vi "MotorMoveIRL.vi"(11 "Rbt Cmd":string) -> (0 "error out":errorcluster)   [LabVIEW 2019]
doc: "Initializes the signals to move the designated motor in the correct direction"
uses:
  <vilib>/myRIO/Instrument Drivers/Onboard IO/DIO/typedefs/DIO Reference.ctl
  <vilib>/myRIO/Common/Instrument Driver Framework/Utilities/typedefs/myRIO Generic Hardware Reference.ctl
  <vilib>/myRIO/Common/Instrument Driver Framework/Utilities/typedefs/Hardware Version Enum.ctl
  <vilib>/myRIO/Common/Instrument Driver Framework/Utilities/typedefs/myRIO v1.0 Reference.ctl
  <vilib>/myRIO/Common/Instrument Driver Framework/Utilities/typedefs/Generic FPGA Reference.ctl
  <vilib>/myRIO/Common/Instrument Driver Framework/myRIO v1.0/DIO/typedefs/DIO Channels List.ctl
  <vilib>/myRIO/Common/Instrument Driver Framework/myRIO v1.0/DIO/typedefs/DIO Channels Enum.ctl
  <vilib>/userDefined/High Color/nirio_resource_hc.ctl
  <vilib>/myRIO/Instrument Drivers/Onboard IO/AO/typedefs/AO Reference.ctl
  <vilib>/myRIO/Common/Instrument Driver Framework/myRIO v1.0/AO/typedefs/AO Channels List.ctl
  <vilib>/myRIO/Common/Instrument Driver Framework/myRIO v1.0/AO/typedefs/AO Channels Enum.ctl
  <vilib>/myRIO/Common/Instrument Driver Framework/Utilities/typedefs/Analog Scaling Constants List.ctl
  <vilib>/myRIO/Common/Instrument Driver Framework/Utilities/typedefs/Analog Scaling Constants.ctl
  <vilib>/myRIO/Common/Instrument Driver Framework/myRIO v1.0/Encoder/typedefs/Encoder Signal Mode.ctl
  <vilib>/myRIO/Instrument Drivers/Onboard IO/Encoder/typedefs/Encoder Reference.ctl
  <vilib>/myRIO/Common/Instrument Driver Framework/myRIO v1.0/Encoder/typedefs/Encoder Channels Enum.ctl
  <vilib>/myRIO/Common/Instrument Driver Framework/myRIO v1.0/Encoder/typedefs/Encoder Configuration v1.0.ctl
  <vilib>/myRIO/Common/Instrument Driver Framework/Utilities/vis/Is FPGA Ref Available.vi
  <vilib>/myRIO/Common/Instrument Driver Framework/myRIO v1.0/DIO/vis/myRIO v1.1 Open DIO.vi
  <vilib>/myRIO/Instrument Drivers/Onboard IO/DIO/vis/Write.vi
  <vilib>/myRIO/Common/Instrument Driver Framework/myRIO v1.0/AO/vis/myRIO v1.1 Open AO.vi
  <vilib>/myRIO/Instrument Drivers/Onboard IO/AO/vis/Write.vi
  <vilib>/myRIO/Common/Instrument Driver Framework/myRIO v1.0/Encoder/vis/myRIO v1.1 Open Encoder.vi
  <vilib>/myRIO/Instrument Drivers/Onboard IO/Encoder/vis/Read.vi
  <vilib>/myRIO/Common/Instrument Driver Framework/Utilities/vis/Validate Channels.vi
  <vilib>/myRIO/Common/Instrument Driver Framework/myRIO v1.0/DIO/vis/myRIO v1.0 Reserve DIO.vi
  <vilib>/myRIO/Common/Instrument Driver Framework/myRIO v1.0/AO/vis/myRIO v1.0 Reserve AO.vi
  <vilib>/myRIO/Common/Instrument Driver Framework/myRIO v1.0/Encoder/vis/myRIO v1.0 Reserve Encoder.vi
  <vilib>/myRIO/Common/Instrument Driver Framework/myRIO v1.0/Resource Manager/vis/myRIO v1.0 Reserve Channel List.vi
  <vilib>/myRIO/Common/Instrument Driver Framework/myRIO v1.0/DIO/vis/myRIO v1.0 Build MUX Configuration DIO.vi
  <vilib>/myRIO/Common/Instrument Driver Framework/myRIO v1.0/AO/vis/myRIO v1.0 Build MUX Configuration AO.vi
  <vilib>/myRIO/Common/Instrument Driver Framework/myRIO v1.0/Encoder/vis/myRIO v1.0 Build MUX Configuration Encoder.vi
  <vilib>/myRIO/Common/Instrument Driver Framework/myRIO v1.0/Resource Manager/vis/myRIO v1.0 Reserve Channel.vi
  <vilib>/myRIO/Common/Instrument Driver Framework/myRIO v1.0/Resource Manager/vis/myRIO v1.0 Unreserve Channel.vi
  <vilib>/myRIO/Common/Instrument Driver Framework/myRIO v1.0/Resource Manager/vis/myRIO v1.0 Create Configuration List.vi
  <vilib>/myRIO/Common/Instrument Driver Framework/myRIO v1.0/Resource Manager/vis/myRIO v1.0 Build Mutex Name.vi
  <vilib>/Utility/VariantDataType/GetNumericInfo.vi
  <vilib>/Utility/error.llb/Error Cluster From Error Code.vi
  <vilib>/myRIO/Common/Instrument Driver Framework/myRIO v1.0/myRIO v1.1 Open.vi
  <vilib>/myRIO/Common/Instrument Driver Framework/Utilities/vis/IO Manager.vi
  <vilib>/myRIO/Common/Instrument Driver Framework/Utilities/vis/Configuration Manager.vi
  <vilib>/myRIO/Common/Instrument Driver Framework/myRIO v1.0/Resource Manager/vis/myRIO v1.0 Configure IO.vi
  <vilib>/myRIO/Common/Instrument Driver Framework/myRIO v1.0/myRIO v1.0 Close.vi
  <vilib>/myRIO/Common/Instrument Driver Framework/myRIO v1.0/DIO/vis/myRIO v1.0 Write DIO.vi
  <vilib>/myRIO/Common/Instrument Driver Framework/myRIO v1.0/AO/vis/myRIO v1.0 Get Scaling Constants AO.vi
  <vilib>/myRIO/Common/Instrument Driver Framework/myRIO v1.0/AO/vis/myRIO v1.0 Write AO.vi
  <vilib>/myRIO/Common/Instrument Driver Framework/myRIO v1.0/Encoder/vis/myRIO v1.0 Configure Encoder.vi
  <vilib>/myRIO/Common/Instrument Driver Framework/myRIO v1.0/Encoder/vis/myRIO v1.0 Read Encoder.vi
  <vilib>/myRIO/Express VI/Onboard IO/DO/DO Express VI.xnode
  <vilib>/myRIO/Instrument Drivers/Onboard IO/DIO/vis/myRIO DIO Open.xnode
  <vilib>/myRIO/Express VI/Onboard IO/AO/AO Express VI.xnode
  <vilib>/myRIO/Instrument Drivers/Onboard IO/AO/vis/myRIO AO Open.xnode
  <vilib>/myRIO/Express VI/Onboard IO/Encoder/Encoder Express VI.xnode
  <vilib>/myRIO/Instrument Drivers/Onboard IO/Encoder/vis/myRIO Encoder Open.xnode
  <vilib>/myRIO/Common/Instrument Driver Framework/myRIO v1.0/Encoder/typedefs/Encoder Count Direction Enum.ctl
  <vilib>/myRIO/Instrument Drivers/Onboard IO/Encoder/Encoder.lvlib
  <vilib>/myRIO/Instrument Drivers/Onboard IO/DIO/DIO.lvlib
  <vilib>/myRIO/Instrument Drivers/Onboard IO/AO/AO.lvlib
panel:
  out "Enco B'":i32
  out "Enco R'":i32
  out "Enco L'":i32
  out "Enco F'":i32
  out "Enco D'":i32
  out "Enco U'":i32
  out "Enco D":i32
  out "Enco U":i32
  out "Enco B":i32
  out "Enco R":i32
  out "Enco L":i32
  out "Enco F":i32
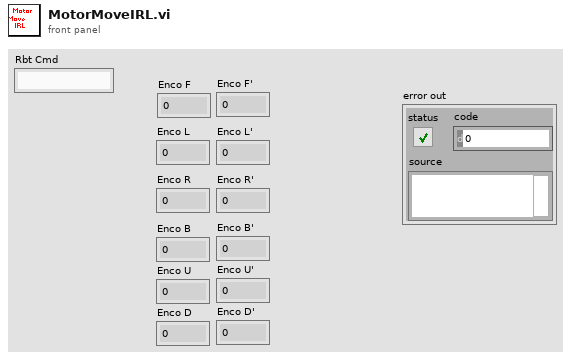
[diagram p1: front panel]
types:
  T1 = typedef "AO.lvlib/AO Reference.ctl" = cluster{"myRIO Reference":T2, "AO Channel List":T6, "AO Scaling Constant List":T8}
  T2 = typedef "myRIO Generic Hardware Reference.ctl" = cluster{"myRIO Model":T3, "myRIO Hardware Reference":T4}
  T3 = typedef "Hardware Version Enum.ctl" = enum16{"Unknown", "myRIO-1900", "myRIO-1950", "roboRIO", "NI ELVIS RIO CM", "ELVIS III"}
  T4 = typedef "myRIO v1.0 Reference.ctl" = cluster{"Generic FPGA Reference":T5, "Allow multiple opens":bool}
  T5 = typedef "Generic FPGA Reference.ctl" = refnum<k20>
  T6 = typedef "AO Channels List.ctl" = T7[]
  T7 = typedef "AO Channels Enum.ctl" = enum16{"Not Connected", "AudioOut/Left", "AudioOut/Right", "C/AO0", "C/AO1", "A/AO0", "A/AO1", "B/AO0", "B/AO1"}
  T8 = typedef "Analog Scaling Constants List.ctl" = T9[]
  T9 = typedef "Analog Scaling Constants.ctl" = cluster{"LSB Weight (Volts)":dbl, "Offset (Volts)":dbl, "Signed?":bool}
  T10 = typedef "nirio_resource_hc.ctl" = tag
  T11 = typedef "Encoder.lvlib/Encoder Reference.ctl" = cluster{"myRIO Reference":T2, "Encoder Channels Enum":T12}
  T12 = typedef "Encoder Channels Enum.ctl" = enum16{"Not Connected", "C/ENC0", "C/ENC1", "A/ENC", "A/ENC0", "A/ENC1", "A/ENC2", "A/ENC3", "A/ENC4", "A/ENC5", "A/ENC6", "A/ENC7", "A/ENC8", "A/ENC9", "B/ENC", "B/ENC0", "B/ENC1", "B/ENC2", "B/ENC3", "B/ENC4", "B/ENC5", "B/ENC6", "B/ENC7", "B/ENC8", "B/ENC9", "DIO/ENC0", "DIO/ENC1", "DIO/ENC2", "DIO/ENC3", "DIO/ENC4"}
  T13 = typedef "Encoder Signal Mode.ctl" = enum16{"Quadrature phase signal", "Step and direction signal"}
  T14 = typedef "DIO.lvlib/DIO Reference.ctl" = cluster{"myRIO Reference":T2, "DIO Channels List":T15}
  T15 = typedef "DIO Channels List.ctl" = T16[]
  T16 = typedef "DIO Channels Enum.ctl" = enum16{"Not Connected", "C/DIO0", "C/DIO1", "C/DIO2", "C/DIO3", "C/DIO4", "C/DIO5", "C/DIO6", "C/DIO7", "A/DIO0", "A/DIO1", "A/DIO2", "A/DIO3", "A/DIO4", "A/DIO5", "A/DIO6", "A/DIO7", "A/DIO8", "A/DIO9", "A/DIO10", "A/DIO11", "A/DIO12", "A/DIO13", "A/DIO14", "A/DIO15", "A/DIO16", "A/DIO17", "A/DIO18", "A/DIO19", "B/DIO0", "B/DIO1", "B/DIO2", "B/DIO3", "B/DIO4", "B/DIO5", "B/DIO6", "B/DIO7", "B/DIO8", "B/DIO9", "B/DIO10", "B/DIO11", "B/DIO12", "B/DIO13", "B/DIO14", "B/DIO15", "B/DIO16", "B/DIO17", "B/DIO18", "B/DIO19", "LED0", "LED1", "LED2", "LED3", "Button0", "DIO/DIO0", "DIO/DIO1", "DIO/DIO2", "DIO/DIO3", "DIO/DIO4", "DIO/DIO5", "DIO/DIO6", "DIO/DIO7", "DIO/DIO8", "DIO/DIO9", "SPI/CS0", "SPI/CS1", "SPI/CS2", "SPI/CS3", "LED RADIO (Green)", "LED RADIO (Red)", "LED COMM (Green)", "LED COMM (Red)", "LED MODE (Green)", "LED MODE (Red)"}
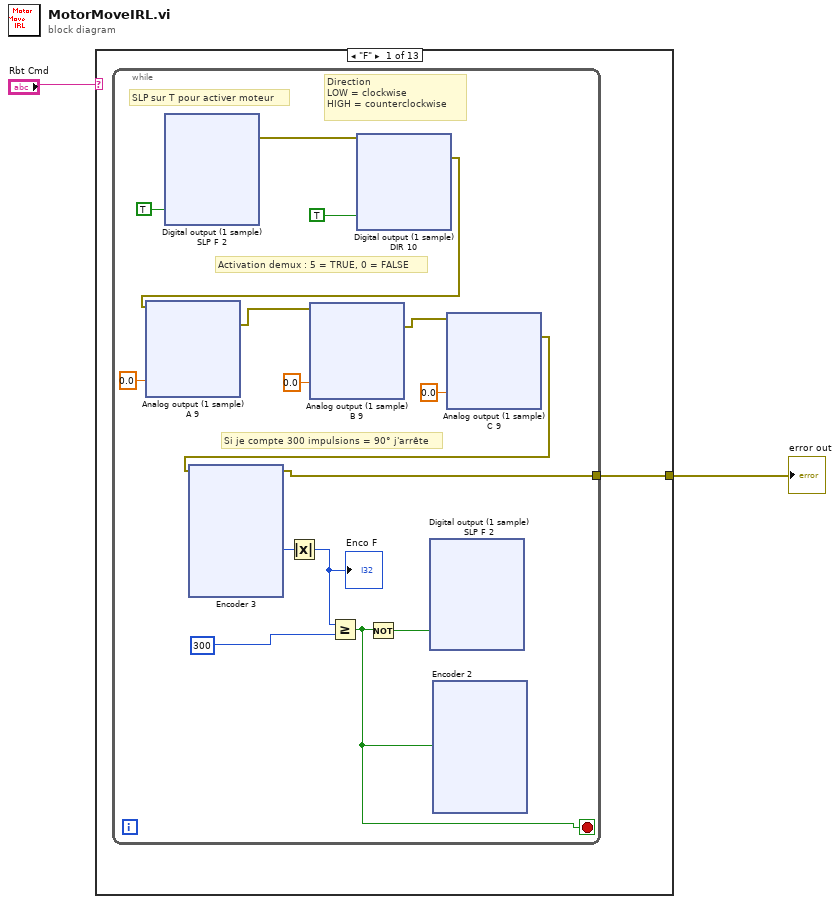
[diagram p0: block diagram]
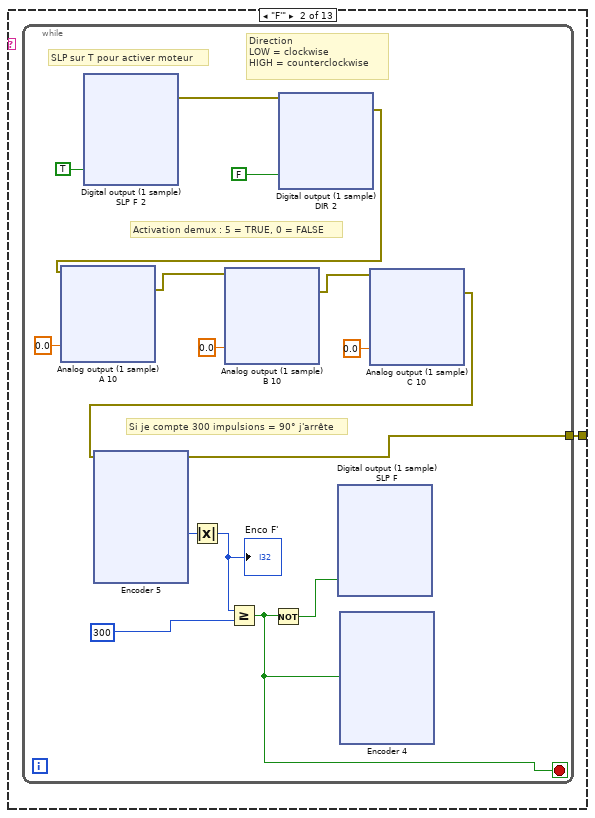
[diagram p2: hidden frame]
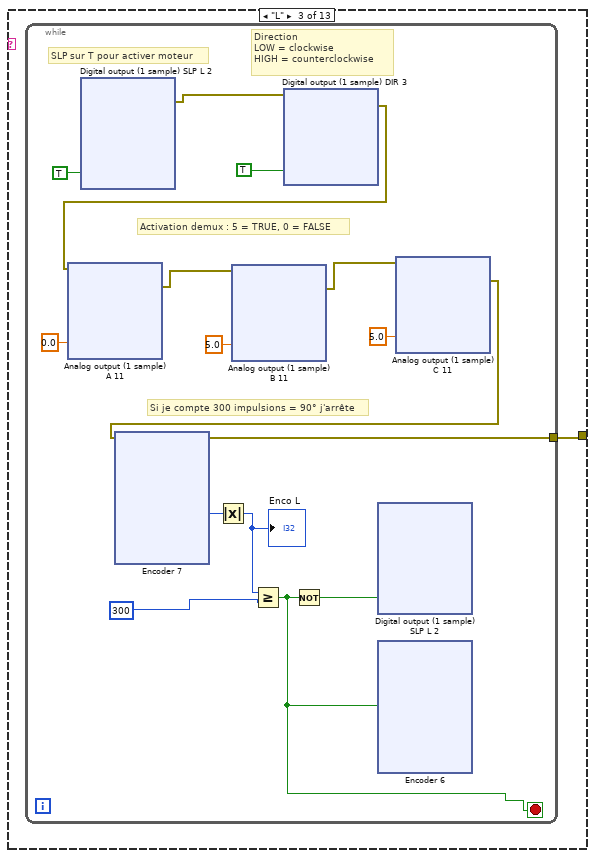
[diagram p3: hidden frame]
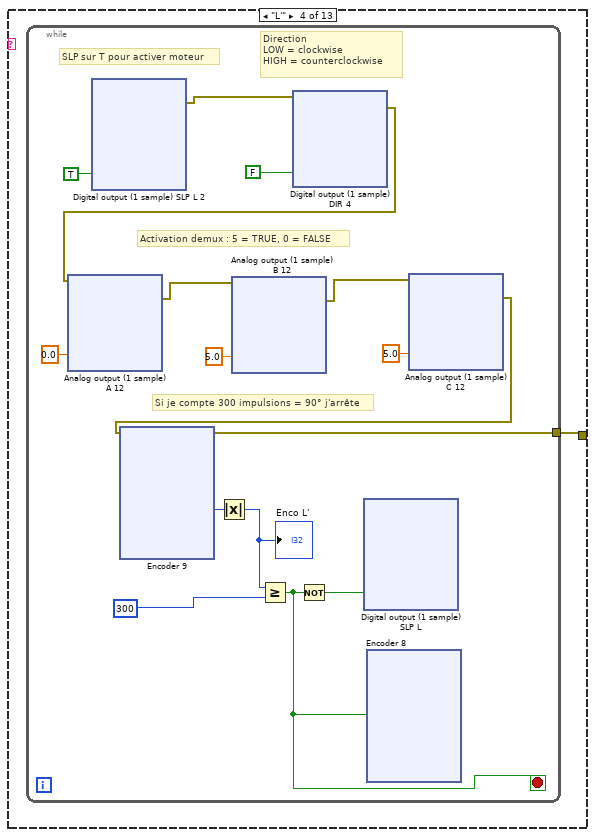
[diagram p4: hidden frame]
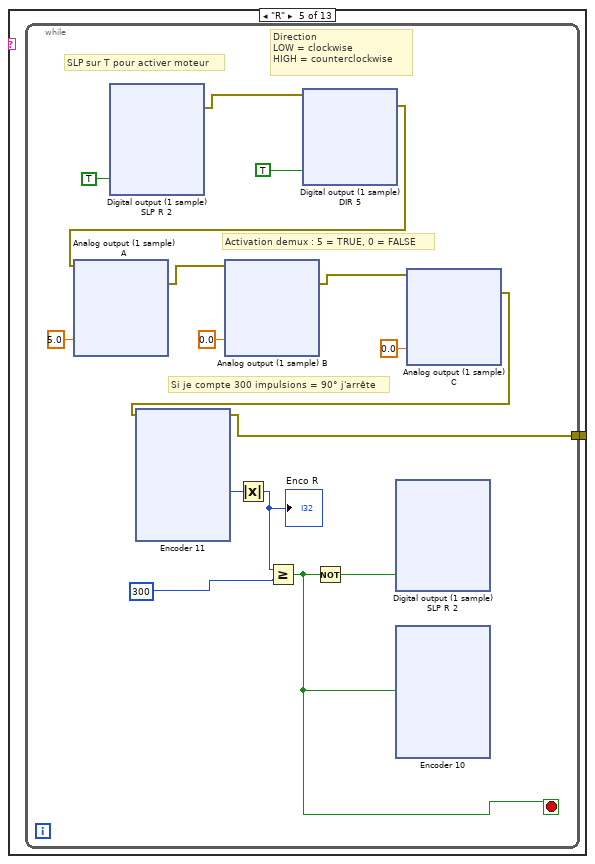
[diagram p5: hidden frame]
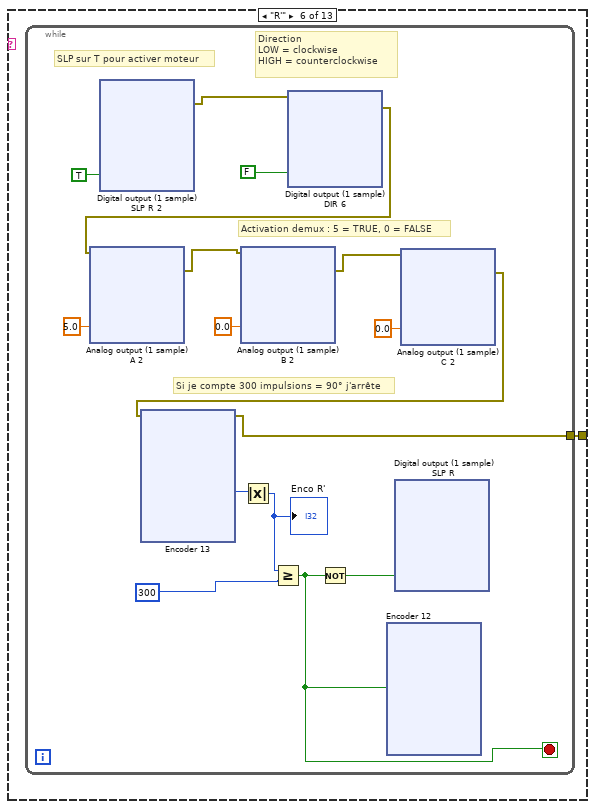
[diagram p6: hidden frame]
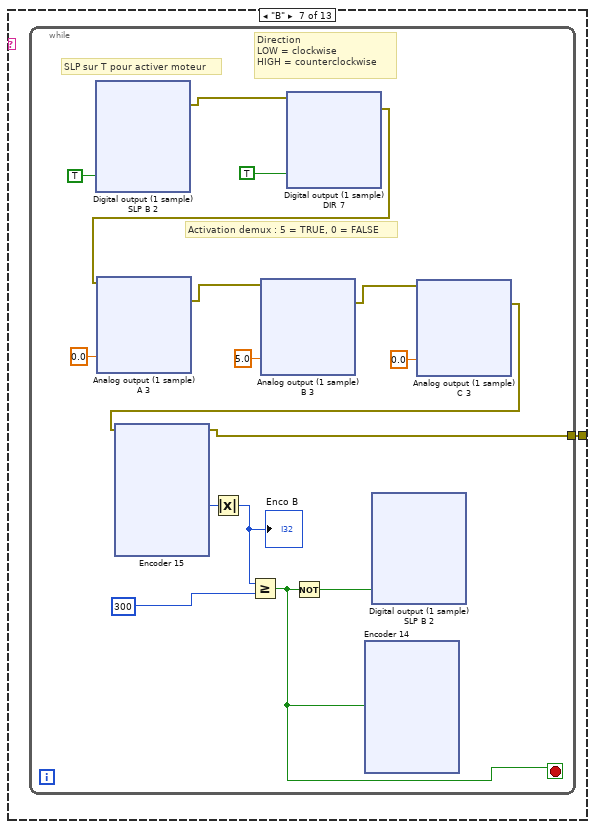
[diagram p7: hidden frame]
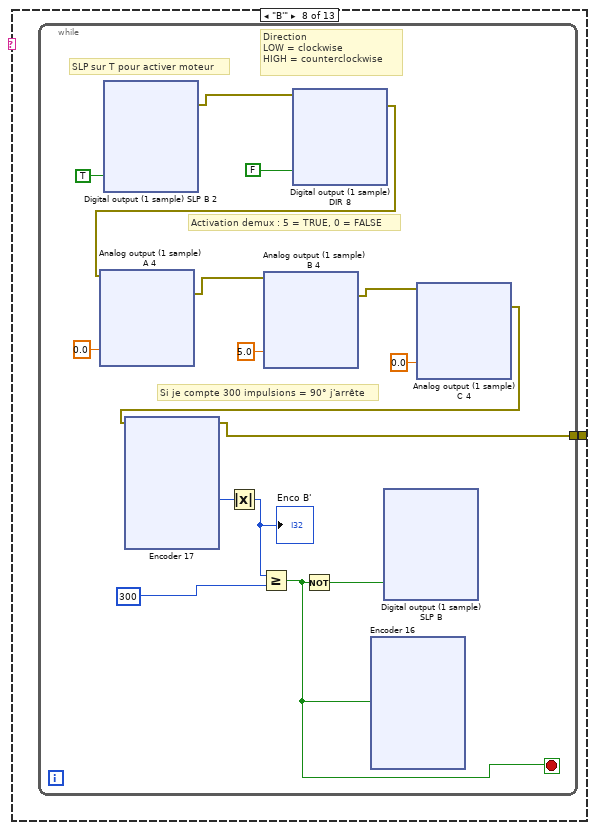
[diagram p8: hidden frame]
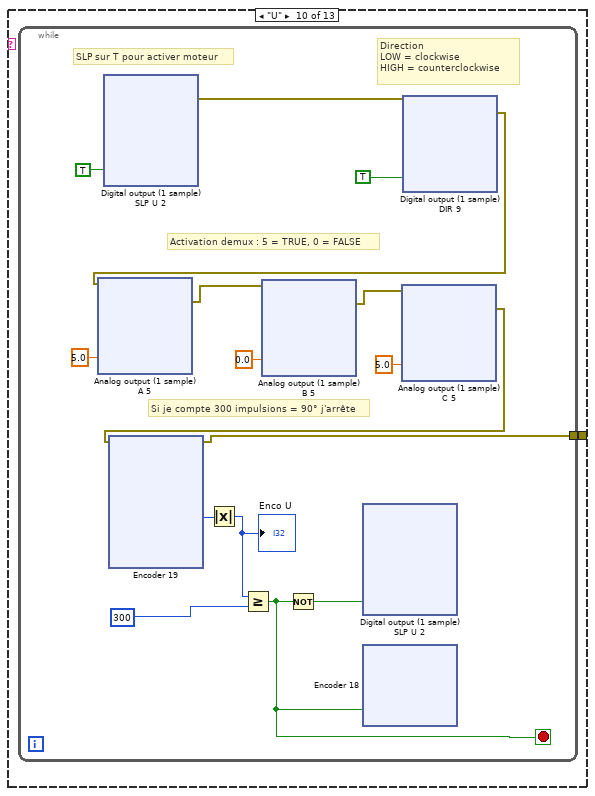
[diagram p10: hidden frame]
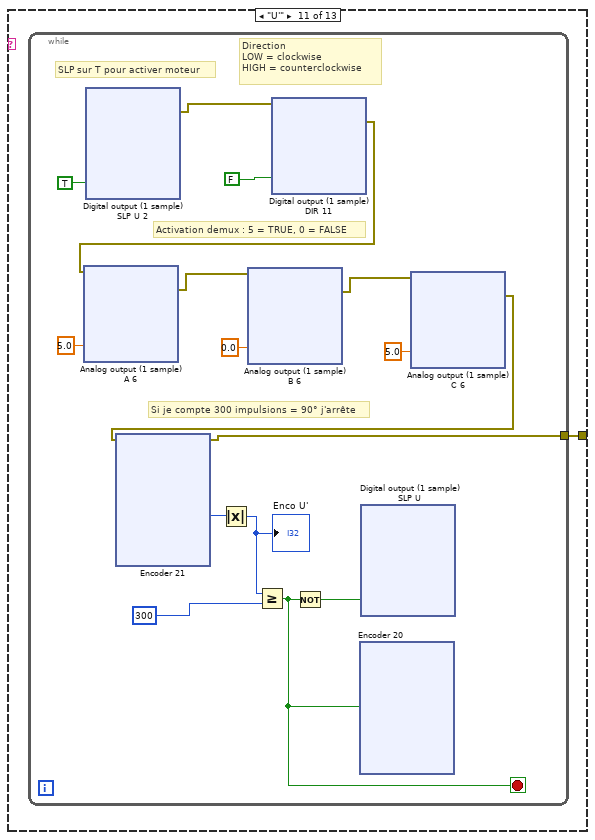
[diagram p11: hidden frame]
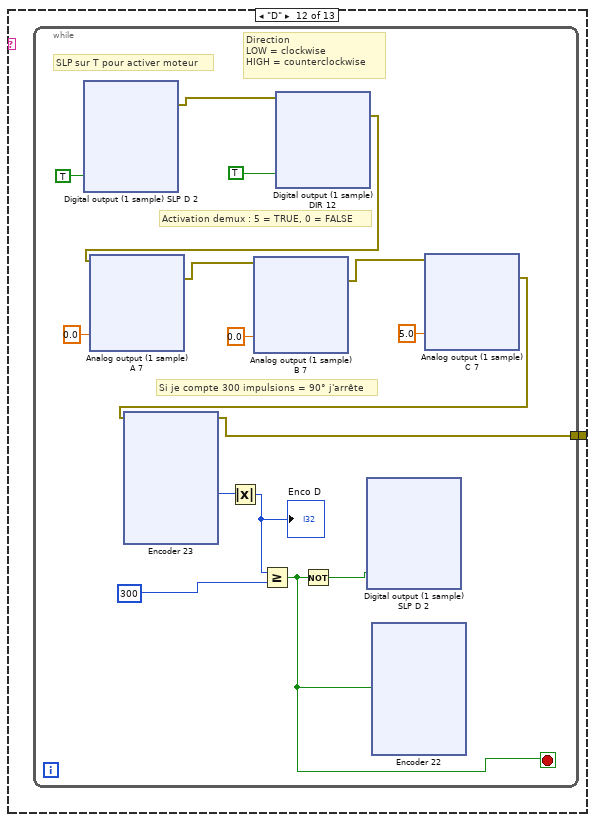
[diagram p12: hidden frame]
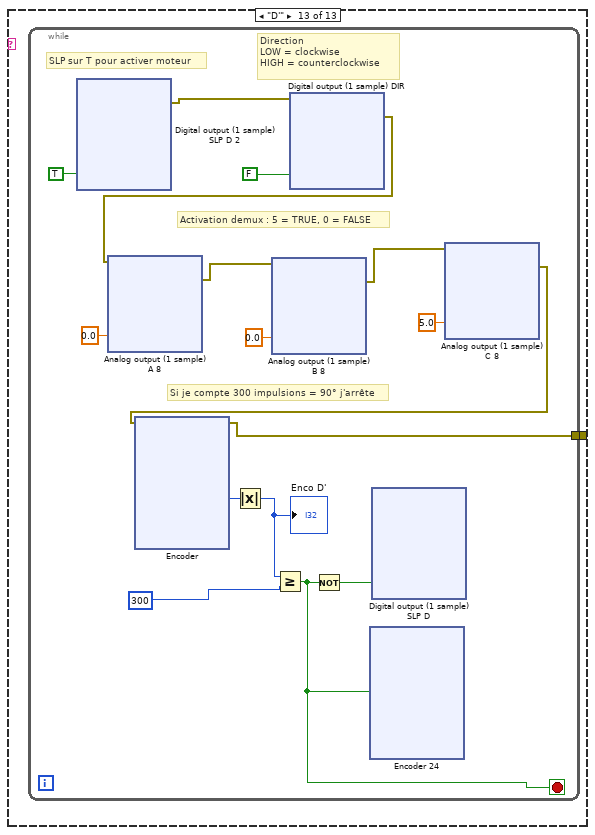
[diagram p13: hidden frame]
diagram:
  n1 = case shown="\"F\"" "Rbt Cmd" {
    tunnel: [w3 w328 w653 w978 w1303 w1628 w1953 w2278 _ w2603 w2928 w3253 w3578] -> w1
    frame "F" {
      n2 = while {
        tunnel: [w4] -> w3
        stop <- w13 stop-if-true
        # "Activation demux : 5 = TRUE, 0 = FALSE"
        # "Si je compte 300 impulsions = 90° j'arrête"
        # "SLP sur T pour activer moteur"
        # "Direction\nLOW = clockwise\nHIGH = counterclockwise"
        n3 = xnode "Digital output (1 sample) SLP F 2"("C/DIO0 (DIO0)"=TRUE) -> ("error out"=w9:errorcluster)  [unwired: 1 in]
        n4 = xnode "Digital output (1 sample) DIR 10"("A/DIO0 (Pin 11)"=TRUE, "error in (no error)"=w9) -> ("error out"=w8:errorcluster)
        n5 = xnode "Analog output (1 sample) A 9"("B/AO0 (Pin 2)"=0.0, "error in (no error)"=w8) -> ("error out"=w7:errorcluster)
        n6 = xnode "Analog output (1 sample) B 9"("B/AO1 (Pin 4)"=0.0, "error in (no error)"=w7) -> ("error out"=w6:errorcluster)
        n7 = xnode "Analog output (1 sample) C 9"("A/AO1 (Pin 4)"=0.0 ("C/AO0 (AO0)"), "error in (no error)"=w6) -> ("error out"=w5:errorcluster)
        n8 = xnode "Encoder 3"("error in (no error)"=w5) -> ("Counter Value"=w15:i32, "error out"=w4:errorcluster)  [unwired: 1 in, 2 out]
        n9 = Absolute Value(x=w15) -> (abs(x)=w16:i32)
        "Enco F" <- w16
        n10 = Greater Or Equal?(x=w16, y=300) -> (x >= y?=w13:bool)
        n11 = Not(x=w13) -> (.not. x?=w17:bool)
        n12 = xnode "Digital output (1 sample) SLP F 2"("C/DIO0 (DIO0)"=w17) -> ()  [unwired: 1 in, 1 out]
        n13 = xnode "Encoder 2"("Reset Counter"=w13) -> ()  [unwired: 1 in, 4 out]
      }
    }
    frame "F'" {
      n14 = while {
        tunnel: [w329] -> w328
        stop <- w343 stop-if-true
        # "Activation demux : 5 = TRUE, 0 = FALSE"
        # "Si je compte 300 impulsions = 90° j'arrête"
        # "SLP sur T pour activer moteur"
        # "Direction\nLOW = clockwise\nHIGH = counterclockwise"
        n15 = xnode "Digital output (1 sample) SLP F 2"("C/DIO0 (DIO0)"=TRUE) -> ("error out"=w334:errorcluster)  [unwired: 1 in]
        n16 = xnode "Digital output (1 sample) DIR 2"("A/DIO0 (Pin 11)"=FALSE, "error in (no error)"=w334) -> ("error out"=w333:errorcluster)
        n17 = xnode "Analog output (1 sample) A 10"("B/AO0 (Pin 2)"=0.0, "error in (no error)"=w333) -> ("error out"=w332:errorcluster)
        n18 = xnode "Analog output (1 sample) B 10"("B/AO1 (Pin 4)"=0.0, "error in (no error)"=w332) -> ("error out"=w331:errorcluster)
        n19 = xnode "Analog output (1 sample) C 10"("A/AO1 (Pin 4)"=0.0 ("C/AO0 (AO0)"), "error in (no error)"=w331) -> ("error out"=w330:errorcluster)
        n20 = xnode "Encoder 5"("error in (no error)"=w330) -> ("Counter Value"=w340:i32, "error out"=w329:errorcluster)  [unwired: 1 in, 2 out]
        n21 = Absolute Value(x=w340) -> (abs(x)=w339:i32)
        "Enco F'" <- w339
        n22 = Greater Or Equal?(x=w339, y=300) -> (x >= y?=w343:bool)
        n23 = Not(x=w343) -> (.not. x?=w341:bool)
        n24 = xnode "Digital output (1 sample) SLP F"("C/DIO0 (DIO0)"=w341) -> ()  [unwired: 1 in, 1 out]
        n25 = xnode "Encoder 4"("Reset Counter"=w343) -> ()  [unwired: 1 in, 4 out]
      }
    }
    frame "L" {
      n26 = while {
        tunnel: [w654] -> w653
        stop <- w668 stop-if-true
        # "Activation demux : 5 = TRUE, 0 = FALSE"
        # "Si je compte 300 impulsions = 90° j'arrête"
        # "SLP sur T pour activer moteur"
        # "Direction\nLOW = clockwise\nHIGH = counterclockwise"
        n27 = xnode "Digital output (1 sample) SLP L 2"("C/DIO3 (DIO3)"=TRUE ("C/DIO0 (DIO0)")) -> ("error out"=w659:errorcluster)  [unwired: 1 in]
        n28 = xnode "Digital output (1 sample) DIR 3"("A/DIO0 (Pin 11)"=TRUE, "error in (no error)"=w659) -> ("error out"=w658:errorcluster)
        n29 = xnode "Analog output (1 sample) A 11"("B/AO0 (Pin 2)"=0.0, "error in (no error)"=w658) -> ("error out"=w657:errorcluster)
        n30 = xnode "Analog output (1 sample) B 11"("B/AO1 (Pin 4)"=5.0, "error in (no error)"=w657) -> ("error out"=w656:errorcluster)
        n31 = xnode "Analog output (1 sample) C 11"("A/AO1 (Pin 4)"=5.0 ("C/AO0 (AO0)"), "error in (no error)"=w656) -> ("error out"=w655:errorcluster)
        n32 = xnode "Encoder 7"("error in (no error)"=w655) -> ("Counter Value"=w665:i32, "error out"=w654:errorcluster)  [unwired: 1 in, 2 out]
        n33 = Absolute Value(x=w665) -> (abs(x)=w664:i32)
        "Enco L" <- w664
        n34 = Greater Or Equal?(x=w664, y=300) -> (x >= y?=w668:bool)
        n35 = Not(x=w668) -> (.not. x?=w666:bool)
        n36 = xnode "Digital output (1 sample) SLP L 2"("C/DIO3 (DIO3)"=w666) -> ()  [unwired: 1 in, 1 out]
        n37 = xnode "Encoder 6"("Reset Counter"=w668) -> ()  [unwired: 1 in, 4 out]
      }
    }
    frame "L'" {
      n38 = while {
        tunnel: [w979] -> w978
        stop <- w993 stop-if-true
        # "Activation demux : 5 = TRUE, 0 = FALSE"
        # "Si je compte 300 impulsions = 90° j'arrête"
        # "SLP sur T pour activer moteur"
        # "Direction\nLOW = clockwise\nHIGH = counterclockwise"
        n39 = xnode "Digital output (1 sample) SLP L 2"("C/DIO3 (DIO3)"=TRUE ("C/DIO0 (DIO0)")) -> ("error out"=w984:errorcluster)  [unwired: 1 in]
        n40 = xnode "Digital output (1 sample) DIR 4"("A/DIO0 (Pin 11)"=FALSE, "error in (no error)"=w984) -> ("error out"=w983:errorcluster)
        n41 = xnode "Analog output (1 sample) A 12"("B/AO0 (Pin 2)"=0.0, "error in (no error)"=w983) -> ("error out"=w982:errorcluster)
        n42 = xnode "Analog output (1 sample) B 12"("B/AO1 (Pin 4)"=5.0, "error in (no error)"=w982) -> ("error out"=w981:errorcluster)
        n43 = xnode "Analog output (1 sample) C 12"("A/AO1 (Pin 4)"=5.0 ("C/AO0 (AO0)"), "error in (no error)"=w981) -> ("error out"=w980:errorcluster)
        n44 = xnode "Encoder 9"("error in (no error)"=w980) -> ("Counter Value"=w989:i32, "error out"=w979:errorcluster)  [unwired: 1 in, 2 out]
        n45 = Absolute Value(x=w989) -> (abs(x)=w990:i32)
        "Enco L'" <- w990
        n46 = Greater Or Equal?(x=w990, y=300) -> (x >= y?=w993:bool)
        n47 = Not(x=w993) -> (.not. x?=w991:bool)
        n48 = xnode "Digital output (1 sample) SLP L"("C/DIO3 (DIO3)"=w991) -> ()  [unwired: 1 in, 1 out]
        n49 = xnode "Encoder 8"("Reset Counter"=w993) -> ()  [unwired: 1 in, 4 out]
      }
    }
    frame "R" {
      n50 = while {
        tunnel: [w1304] -> w1303
        stop <- w1318 stop-if-true
        # "Si je compte 300 impulsions = 90° j'arrête"
        # "SLP sur T pour activer moteur"
        # "Activation demux : 5 = TRUE, 0 = FALSE"
        # "Direction\nLOW = clockwise\nHIGH = counterclockwise"
        n51 = xnode "Digital output (1 sample) SLP R 2"("C/DIO1 (DIO1)"=TRUE ("C/DIO0 (DIO0)")) -> ("error out"=w1309:errorcluster)  [unwired: 1 in]
        n52 = xnode "Digital output (1 sample) DIR 5"("A/DIO0 (Pin 11)"=TRUE, "error in (no error)"=w1309) -> ("error out"=w1308:errorcluster)
        n53 = xnode "Analog output (1 sample) A"("B/AO0 (Pin 2)"=5.0, "error in (no error)"=w1308) -> ("error out"=w1307:errorcluster)
        n54 = xnode "Analog output (1 sample) B"("B/AO1 (Pin 4)"=0.0, "error in (no error)"=w1307) -> ("error out"=w1306:errorcluster)
        n55 = xnode "Analog output (1 sample) C"("A/AO1 (Pin 4)"=0.0 ("C/AO0 (AO0)"), "error in (no error)"=w1306) -> ("error out"=w1305:errorcluster)
        n56 = xnode "Encoder 11"("error in (no error)"=w1305) -> ("Counter Value"=w1315:i32, "error out"=w1304:errorcluster)  [unwired: 1 in, 2 out]
        n57 = Absolute Value(x=w1315) -> (abs(x)=w1314:i32)
        "Enco R" <- w1314
        n58 = Greater Or Equal?(x=w1314, y=300) -> (x >= y?=w1318:bool)
        n59 = Not(x=w1318) -> (.not. x?=w1316:bool)
        n60 = xnode "Digital output (1 sample) SLP R 2"("C/DIO1 (DIO1)"=w1316) -> ()  [unwired: 1 in, 1 out]
        n61 = xnode "Encoder 10"("Reset Counter"=w1318) -> ()  [unwired: 1 in, 4 out]
      }
    }
    frame "R'" {
      n62 = while {
        tunnel: [w1629] -> w1628
        stop <- w1643 stop-if-true
        # "Activation demux : 5 = TRUE, 0 = FALSE"
        # "Si je compte 300 impulsions = 90° j'arrête"
        # "SLP sur T pour activer moteur"
        # "Direction\nLOW = clockwise\nHIGH = counterclockwise"
        n63 = xnode "Digital output (1 sample) SLP R 2"("C/DIO1 (DIO1)"=TRUE ("C/DIO0 (DIO0)")) -> ("error out"=w1634:errorcluster)  [unwired: 1 in]
        n64 = xnode "Digital output (1 sample) DIR 6"("A/DIO0 (Pin 11)"=FALSE, "error in (no error)"=w1634) -> ("error out"=w1633:errorcluster)
        n65 = xnode "Analog output (1 sample) A 2"("B/AO0 (Pin 2)"=5.0, "error in (no error)"=w1633) -> ("error out"=w1632:errorcluster)
        n66 = xnode "Analog output (1 sample) B 2"("B/AO1 (Pin 4)"=0.0, "error in (no error)"=w1632) -> ("error out"=w1631:errorcluster)
        n67 = xnode "Analog output (1 sample) C 2"("A/AO1 (Pin 4)"=0.0 ("C/AO0 (AO0)"), "error in (no error)"=w1631) -> ("error out"=w1630:errorcluster)
        n68 = xnode "Encoder 13"("error in (no error)"=w1630) -> ("Counter Value"=w1640:i32, "error out"=w1629:errorcluster)  [unwired: 1 in, 2 out]
        n69 = Absolute Value(x=w1640) -> (abs(x)=w1639:i32)
        "Enco R'" <- w1639
        n70 = Greater Or Equal?(x=w1639, y=300) -> (x >= y?=w1643:bool)
        n71 = Not(x=w1643) -> (.not. x?=w1641:bool)
        n72 = xnode "Encoder 12"("Reset Counter"=w1643) -> ()  [unwired: 1 in, 4 out]
        n73 = xnode "Digital output (1 sample) SLP R"("C/DIO1 (DIO1)"=w1641) -> ()  [unwired: 1 in, 1 out]
      }
    }
    frame "B" {
      n74 = while {
        tunnel: [w1954] -> w1953
        stop <- w1968 stop-if-true
        # "Activation demux : 5 = TRUE, 0 = FALSE"
        # "SLP sur T pour activer moteur"
        # "Direction\nLOW = clockwise\nHIGH = counterclockwise"
        n75 = xnode "Digital output (1 sample) SLP B 2"("C/DIO2 (DIO2)"=TRUE ("C/DIO0 (DIO0)")) -> ("error out"=w1959:errorcluster)  [unwired: 1 in]
        n76 = xnode "Digital output (1 sample) DIR 7"("A/DIO0 (Pin 11)"=TRUE, "error in (no error)"=w1959) -> ("error out"=w1958:errorcluster)
        n77 = xnode "Analog output (1 sample) A 3"("B/AO0 (Pin 2)"=0.0, "error in (no error)"=w1958) -> ("error out"=w1957:errorcluster)
        n78 = xnode "Analog output (1 sample) B 3"("B/AO1 (Pin 4)"=5.0, "error in (no error)"=w1957) -> ("error out"=w1956:errorcluster)
        n79 = xnode "Analog output (1 sample) C 3"("A/AO1 (Pin 4)"=0.0 ("C/AO0 (AO0)"), "error in (no error)"=w1956) -> ("error out"=w1955:errorcluster)
        n80 = xnode "Encoder 15"("error in (no error)"=w1955) -> ("Counter Value"=w1964:i32, "error out"=w1954:errorcluster)  [unwired: 1 in, 2 out]
        n81 = Absolute Value(x=w1964) -> (abs(x)=w1965:i32)
        "Enco B" <- w1965
        n82 = Greater Or Equal?(x=w1965, y=300) -> (x >= y?=w1968:bool)
        n83 = Not(x=w1968) -> (.not. x?=w1966:bool)
        n84 = xnode "Encoder 14"("Reset Counter"=w1968) -> ()  [unwired: 1 in, 4 out]
        n85 = xnode "Digital output (1 sample) SLP B 2"("C/DIO2 (DIO2)"=w1966) -> ()  [unwired: 1 in, 1 out]
      }
    }
    frame "B'" {
      n86 = while {
        tunnel: [w2279] -> w2278
        stop <- w2293 stop-if-true
        # "Activation demux : 5 = TRUE, 0 = FALSE"
        # "Si je compte 300 impulsions = 90° j'arrête"
        # "SLP sur T pour activer moteur"
        # "Direction\nLOW = clockwise\nHIGH = counterclockwise"
        n87 = xnode "Digital output (1 sample) SLP B 2"("C/DIO2 (DIO2)"=TRUE ("C/DIO0 (DIO0)")) -> ("error out"=w2284:errorcluster)  [unwired: 1 in]
        n88 = xnode "Digital output (1 sample) DIR 8"("A/DIO0 (Pin 11)"=FALSE, "error in (no error)"=w2284) -> ("error out"=w2283:errorcluster)
        n89 = xnode "Analog output (1 sample) A 4"("B/AO0 (Pin 2)"=0.0, "error in (no error)"=w2283) -> ("error out"=w2282:errorcluster)
        n90 = xnode "Analog output (1 sample) B 4"("B/AO1 (Pin 4)"=5.0, "error in (no error)"=w2282) -> ("error out"=w2281:errorcluster)
        n91 = xnode "Analog output (1 sample) C 4"("A/AO1 (Pin 4)"=0.0 ("C/AO0 (AO0)"), "error in (no error)"=w2281) -> ("error out"=w2280:errorcluster)
        n92 = xnode "Encoder 17"("error in (no error)"=w2280) -> ("Counter Value"=w2290:i32, "error out"=w2279:errorcluster)  [unwired: 1 in, 2 out]
        n93 = Absolute Value(x=w2290) -> (abs(x)=w2289:i32)
        "Enco B'" <- w2289
        n94 = Greater Or Equal?(x=w2289, y=300) -> (x >= y?=w2293:bool)
        n95 = Not(x=w2293) -> (.not. x?=w2291:bool)
        n96 = xnode "Encoder 16"("Reset Counter"=w2293) -> ()  [unwired: 1 in, 4 out]
        n97 = xnode "Digital output (1 sample) SLP B"("C/DIO2 (DIO2)"=w2291) -> ()  [unwired: 1 in, 1 out]
      }
    }
    frame "", Default {
    }
    frame "U" {
      n98 = while {
        tunnel: [w2604] -> w2603
        stop <- w2618 stop-if-true
        # "Activation demux : 5 = TRUE, 0 = FALSE"
        # "Si je compte 300 impulsions = 90° j'arrête"
        # "SLP sur T pour activer moteur"
        # "Direction\nLOW = clockwise\nHIGH = counterclockwise"
        n99 = xnode "Digital output (1 sample) SLP U 2"("C/DIO5 (DIO5)"=TRUE ("C/DIO0 (DIO0)")) -> ("error out"=w2609:errorcluster)  [unwired: 1 in]
        n100 = xnode "Digital output (1 sample) DIR 9"("A/DIO0 (Pin 11)"=TRUE, "error in (no error)"=w2609) -> ("error out"=w2608:errorcluster)
        n101 = xnode "Analog output (1 sample) A 5"("B/AO0 (Pin 2)"=5.0, "error in (no error)"=w2608) -> ("error out"=w2607:errorcluster)
        n102 = xnode "Analog output (1 sample) B 5"("B/AO1 (Pin 4)"=0.0, "error in (no error)"=w2607) -> ("error out"=w2606:errorcluster)
        n103 = xnode "Analog output (1 sample) C 5"("A/AO1 (Pin 4)"=5.0 ("C/AO0 (AO0)"), "error in (no error)"=w2606) -> ("error out"=w2605:errorcluster)
        n104 = xnode "Encoder 19"("error in (no error)"=w2605) -> ("Counter Value"=w2614:i32, "error out"=w2604:errorcluster)  [unwired: 1 in, 2 out]
        n105 = Absolute Value(x=w2614) -> (abs(x)=w2613:i32)
        "Enco U" <- w2613
        n106 = Greater Or Equal?(x=w2613, y=300) -> (x >= y?=w2618:bool)
        n107 = Not(x=w2618) -> (.not. x?=w2616:bool)
        n108 = xnode "Digital output (1 sample) SLP U 2"("C/DIO5 (DIO5)"=w2616) -> ()  [unwired: 1 in, 1 out]
        n109 = xnode "Encoder 18"("Reset Counter"=w2618) -> ()  [unwired: 1 in, 4 out]
      }
    }
    frame "U'" {
      n110 = while {
        tunnel: [w2929] -> w2928
        stop <- w2943 stop-if-true
        # "Activation demux : 5 = TRUE, 0 = FALSE"
        # "Si je compte 300 impulsions = 90° j'arrête"
        # "SLP sur T pour activer moteur"
        # "Direction\nLOW = clockwise\nHIGH = counterclockwise"
        n111 = xnode "Digital output (1 sample) SLP U 2"("C/DIO5 (DIO5)"=TRUE ("C/DIO0 (DIO0)")) -> ("error out"=w2934:errorcluster)  [unwired: 1 in]
        n112 = xnode "Digital output (1 sample) DIR 11"("A/DIO0 (Pin 11)"=FALSE, "error in (no error)"=w2934) -> ("error out"=w2933:errorcluster)
        n113 = xnode "Analog output (1 sample) A 6"("B/AO0 (Pin 2)"=5.0, "error in (no error)"=w2933) -> ("error out"=w2932:errorcluster)
        n114 = xnode "Analog output (1 sample) B 6"("B/AO1 (Pin 4)"=0.0, "error in (no error)"=w2932) -> ("error out"=w2931:errorcluster)
        n115 = xnode "Analog output (1 sample) C 6"("A/AO1 (Pin 4)"=5.0 ("C/AO0 (AO0)"), "error in (no error)"=w2931) -> ("error out"=w2930:errorcluster)
        n116 = xnode "Encoder 21"("error in (no error)"=w2930) -> ("Counter Value"=w2938:i32, "error out"=w2929:errorcluster)  [unwired: 1 in, 2 out]
        n117 = Absolute Value(x=w2938) -> (abs(x)=w2939:i32)
        "Enco U'" <- w2939
        n118 = Greater Or Equal?(x=w2939, y=300) -> (x >= y?=w2943:bool)
        n119 = Not(x=w2943) -> (.not. x?=w2941:bool)
        n120 = xnode "Encoder 20"("Reset Counter"=w2943) -> ()  [unwired: 1 in, 4 out]
        n121 = xnode "Digital output (1 sample) SLP U"("C/DIO5 (DIO5)"=w2941) -> ()  [unwired: 1 in, 1 out]
      }
    }
    frame "D" {
      n122 = while {
        tunnel: [w3254] -> w3253
        stop <- w3268 stop-if-true
        # "Activation demux : 5 = TRUE, 0 = FALSE"
        # "Si je compte 300 impulsions = 90° j'arrête"
        # "SLP sur T pour activer moteur"
        # "Direction\nLOW = clockwise\nHIGH = counterclockwise"
        n123 = xnode "Digital output (1 sample) SLP D 2"("C/DIO4 (DIO4)"=TRUE ("C/DIO0 (DIO0)")) -> ("error out"=w3259:errorcluster)  [unwired: 1 in]
        n124 = xnode "Digital output (1 sample) DIR 12"("A/DIO0 (Pin 11)"=TRUE, "error in (no error)"=w3259) -> ("error out"=w3258:errorcluster)
        n125 = xnode "Analog output (1 sample) A 7"("B/AO0 (Pin 2)"=0.0, "error in (no error)"=w3258) -> ("error out"=w3257:errorcluster)
        n126 = xnode "Analog output (1 sample) B 7"("B/AO1 (Pin 4)"=0.0, "error in (no error)"=w3257) -> ("error out"=w3256:errorcluster)
        n127 = xnode "Analog output (1 sample) C 7"("A/AO1 (Pin 4)"=5.0 ("C/AO0 (AO0)"), "error in (no error)"=w3256) -> ("error out"=w3255:errorcluster)
        n128 = xnode "Encoder 23"("error in (no error)"=w3255) -> ("Counter Value"=w3265:i32, "error out"=w3254:errorcluster)  [unwired: 1 in, 2 out]
        n129 = Absolute Value(x=w3265) -> (abs(x)=w3264:i32)
        "Enco D" <- w3264
        n130 = Greater Or Equal?(x=w3264, y=300) -> (x >= y?=w3268:bool)
        n131 = Not(x=w3268) -> (.not. x?=w3266:bool)
        n132 = xnode "Digital output (1 sample) SLP D 2"("C/DIO4 (DIO4)"=w3266) -> ()  [unwired: 1 in, 1 out]
        n133 = xnode "Encoder 22"("Reset Counter"=w3268) -> ()  [unwired: 1 in, 4 out]
      }
    }
    frame "D'" {
      n134 = while {
        tunnel: [w3579] -> w3578
        stop <- w3593 stop-if-true
        # "Activation demux : 5 = TRUE, 0 = FALSE"
        # "Si je compte 300 impulsions = 90° j'arrête"
        # "SLP sur T pour activer moteur"
        # "Direction\nLOW = clockwise\nHIGH = counterclockwise"
        n135 = xnode "Digital output (1 sample) SLP D 2"("C/DIO4 (DIO4)"=TRUE ("C/DIO0 (DIO0)")) -> ("error out"=w3584:errorcluster)  [unwired: 1 in]
        n136 = xnode "Digital output (1 sample) DIR"("A/DIO0 (Pin 11)"=FALSE, "error in (no error)"=w3584) -> ("error out"=w3583:errorcluster)
        n137 = xnode "Analog output (1 sample) A 8"("B/AO0 (Pin 2)"=0.0, "error in (no error)"=w3583) -> ("error out"=w3582:errorcluster)
        n138 = xnode "Analog output (1 sample) B 8"("B/AO1 (Pin 4)"=0.0, "error in (no error)"=w3582) -> ("error out"=w3581:errorcluster)
        n139 = xnode "Analog output (1 sample) C 8"("A/AO1 (Pin 4)"=5.0 ("C/AO0 (AO0)"), "error in (no error)"=w3581) -> ("error out"=w3580:errorcluster)
        n140 = xnode "Encoder"("error in (no error)"=w3580) -> ("Counter Value"=w3590:i32, "error out"=w3579:errorcluster)  [unwired: 1 in, 2 out]
        n141 = Absolute Value(x=w3590) -> (abs(x)=w3589:i32)
        "Enco D'" <- w3589
        n142 = Greater Or Equal?(x=w3589, y=300) -> (x >= y?=w3593:bool)
        n143 = Not(x=w3593) -> (.not. x?=w3591:bool)
        n144 = xnode "Encoder 24"("Reset Counter"=w3593) -> ()  [unwired: 1 in, 4 out]
        n145 = xnode "Digital output (1 sample) SLP D"("C/DIO4 (DIO4)"=w3591) -> ()  [unwired: 1 in, 1 out]
      }
    }
  }
  "error out" <- w1
